vi "DBDeleteRecord.vi"(8 "error in (no error)":errorcluster, 9 "message value":variant, 11 "ProcessState in":T1) -> (0 "error out":errorcluster, 3 "ProcessState out":T1)   [LabVIEW 2015, in "FileHandler.lvlib"]
uses:
  FileHandler.lvlib
  controls/ProcessState.ctl
  <vilib>/drjdpowell/SQLite Library/SQL Connection/Connection.lvclass
  <vilib>/drjdpowell/SQLite Library/SQL Statement/SQL Statement.lvclass/SQL Statement.ctl
  <vilib>/drjdpowell/SQLite Library/SQL Statement/Bind Timestamp (Text).vi
  <vilib>/drjdpowell/SQLite Library/SQL Statement/Bind Text.vi
  <vilib>/drjdpowell/SQLite Library/SQL Statement/Error Message.vi
  DBToolkit/DBToolkit.lvlib
  <vilib>/drjdpowell/SQLite Library/SQL Statement/SQL Statement.lvclass
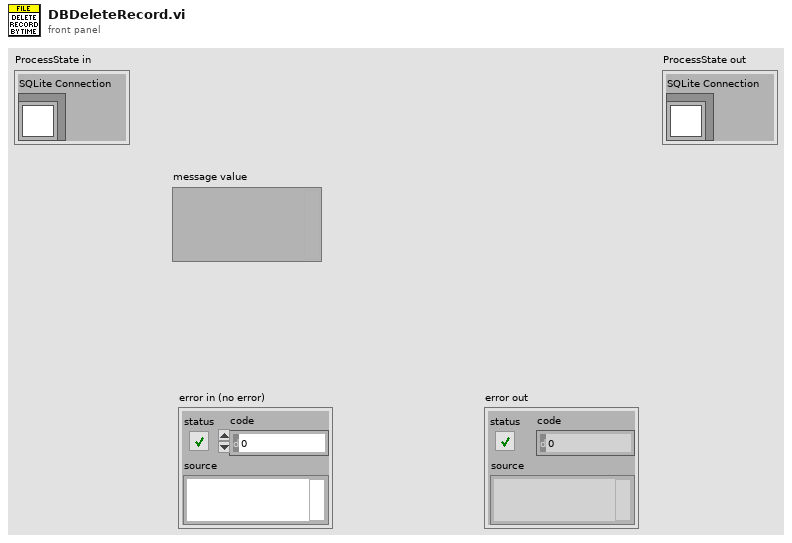
[diagram p1: front panel]
types:
  T1 = typedef "FileHandler.lvlib/ProcessState.ctl" = cluster{"SQLite Connection":refnum<class "Connection.lvclass">}
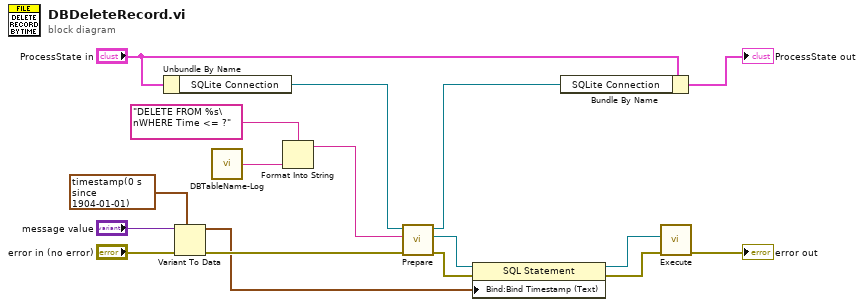
[diagram p0: block diagram]
diagram:
  n1 = Unbundle By Name("ProcessState in") -> ("SQLite Connection"=w12:refnum<class "Connection.lvclass">)
  n2 = Variant To Data(error in="error in (no error)", type=timestamp(0 s since 1904-01-01), Variant="message value") -> (data=w1:timestamp, error out=w13:errorcluster)
  n3 = call "DBTableName-Log.vi"() -> ("DB Table Name"=w4:string)  [unwired: 5 in]
  n4 = Format Into String(format string="DELETE FROM %s\nWHERE Time <= ?", w4) -> (resulting string=w3:string)  [unwired: 2 in, 1 out]
  n5 = call <vilib>:"Prepare.vi"("error in (no error)"=w13, "SQL"=w3, "SQLite Connection in"=w12) -> ("error out"=w11:errorcluster, "SQL Statement out"=w10:refnum<class "SQL Statement.lvclass">, "SQLite Connection out"=w6:refnum<class "Connection.lvclass">)  [unwired: 4 in, 2 out]
  n6 = property class="SQL Statement"(reference=w10, error in=w11, "Bind:Bind Timestamp (Text)"=w1) -> (reference out=w9:refnum<class "SQL Statement.lvclass">, error out=w8:errorcluster)
  n7 = Bundle By Name(cluster="ProcessState in", "SQLite Connection"=w6) -> (→"ProcessState out":T1)
  n8 = call "Execute.vi"("error in (no error)"=w8, "SQL Statement in"=w9) -> ("error out"=→"error out":errorcluster)  [unwired: 9 in]
